vi "SetOutSumvGainAndOffset.vi"(6 "time out":u32, 9 "Real1":dbl, 10 "类型":u32(ring)=4 items=["PCI5121"=1, "PCI9810"=2, "USBCAN1"=3, "USBCAN2"=4, "PCI9820"=5, "CAN232"=6, "PCI5110"=7, "CANLite(mini)"=8, "ISA9620"=9, "ISA5420"=10, "PC104CAN"=11, "CANET"=17, "DNP9810"=13, "USBCAN-E-U"=20, "USBCAN-2E-U"=21], 11 "Real2":dbl, 12 "设备索引":u32(ring) items=["0", "1", "2", "3", "4", "5", "6", "7", "8", "9", "10", "11", "12", "13", "14", "15", ""], 13 "AD1":u16, 15 "AD2":u16, 16 "CAN路数":u32(ring) items=["0", "1"]) -> (20 "set ok?":bool, 22 "Gain":u16, 23 "Offset":u32)   [LabVIEW 2013]
uses:
  AutoBurn/Settings/ControlCAN.dll
panel:
  out "VCI_CAN_OBJ_T":T1 {"ID" format="%x"}
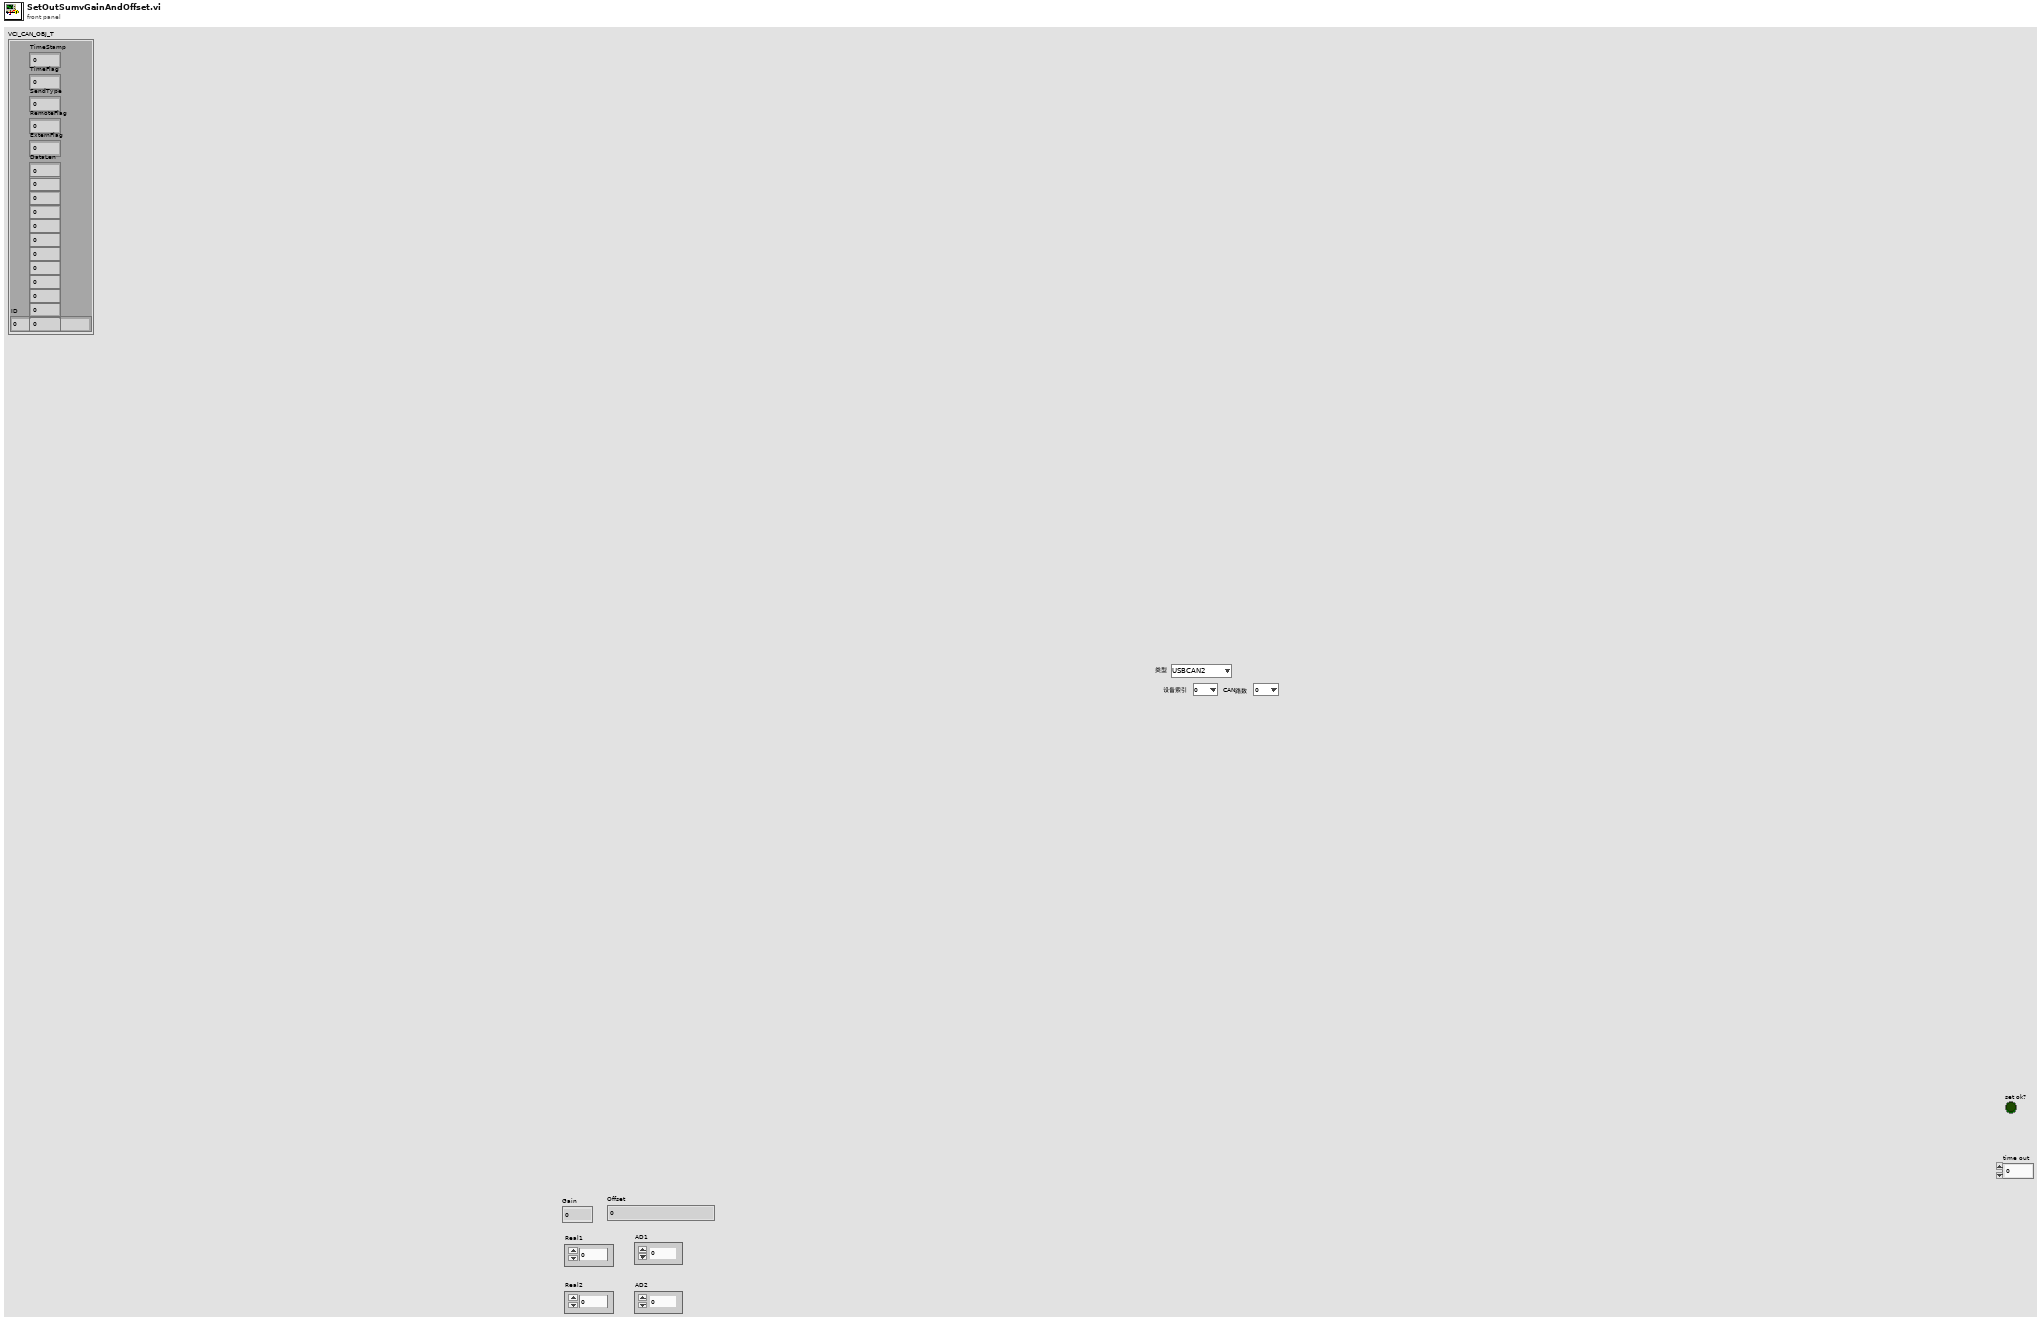
[diagram p1: front panel]
types:
  T1 = cluster{"ID":u32, "TimeStamp":u32, "TimeFlag":u8, "SendType":u8, "RemoteFlag":u8, "ExternFlag":u8, "DataLen":u8, u8, u8, u8, u8, u8, u8, u8, u8, u8, u8, u8}
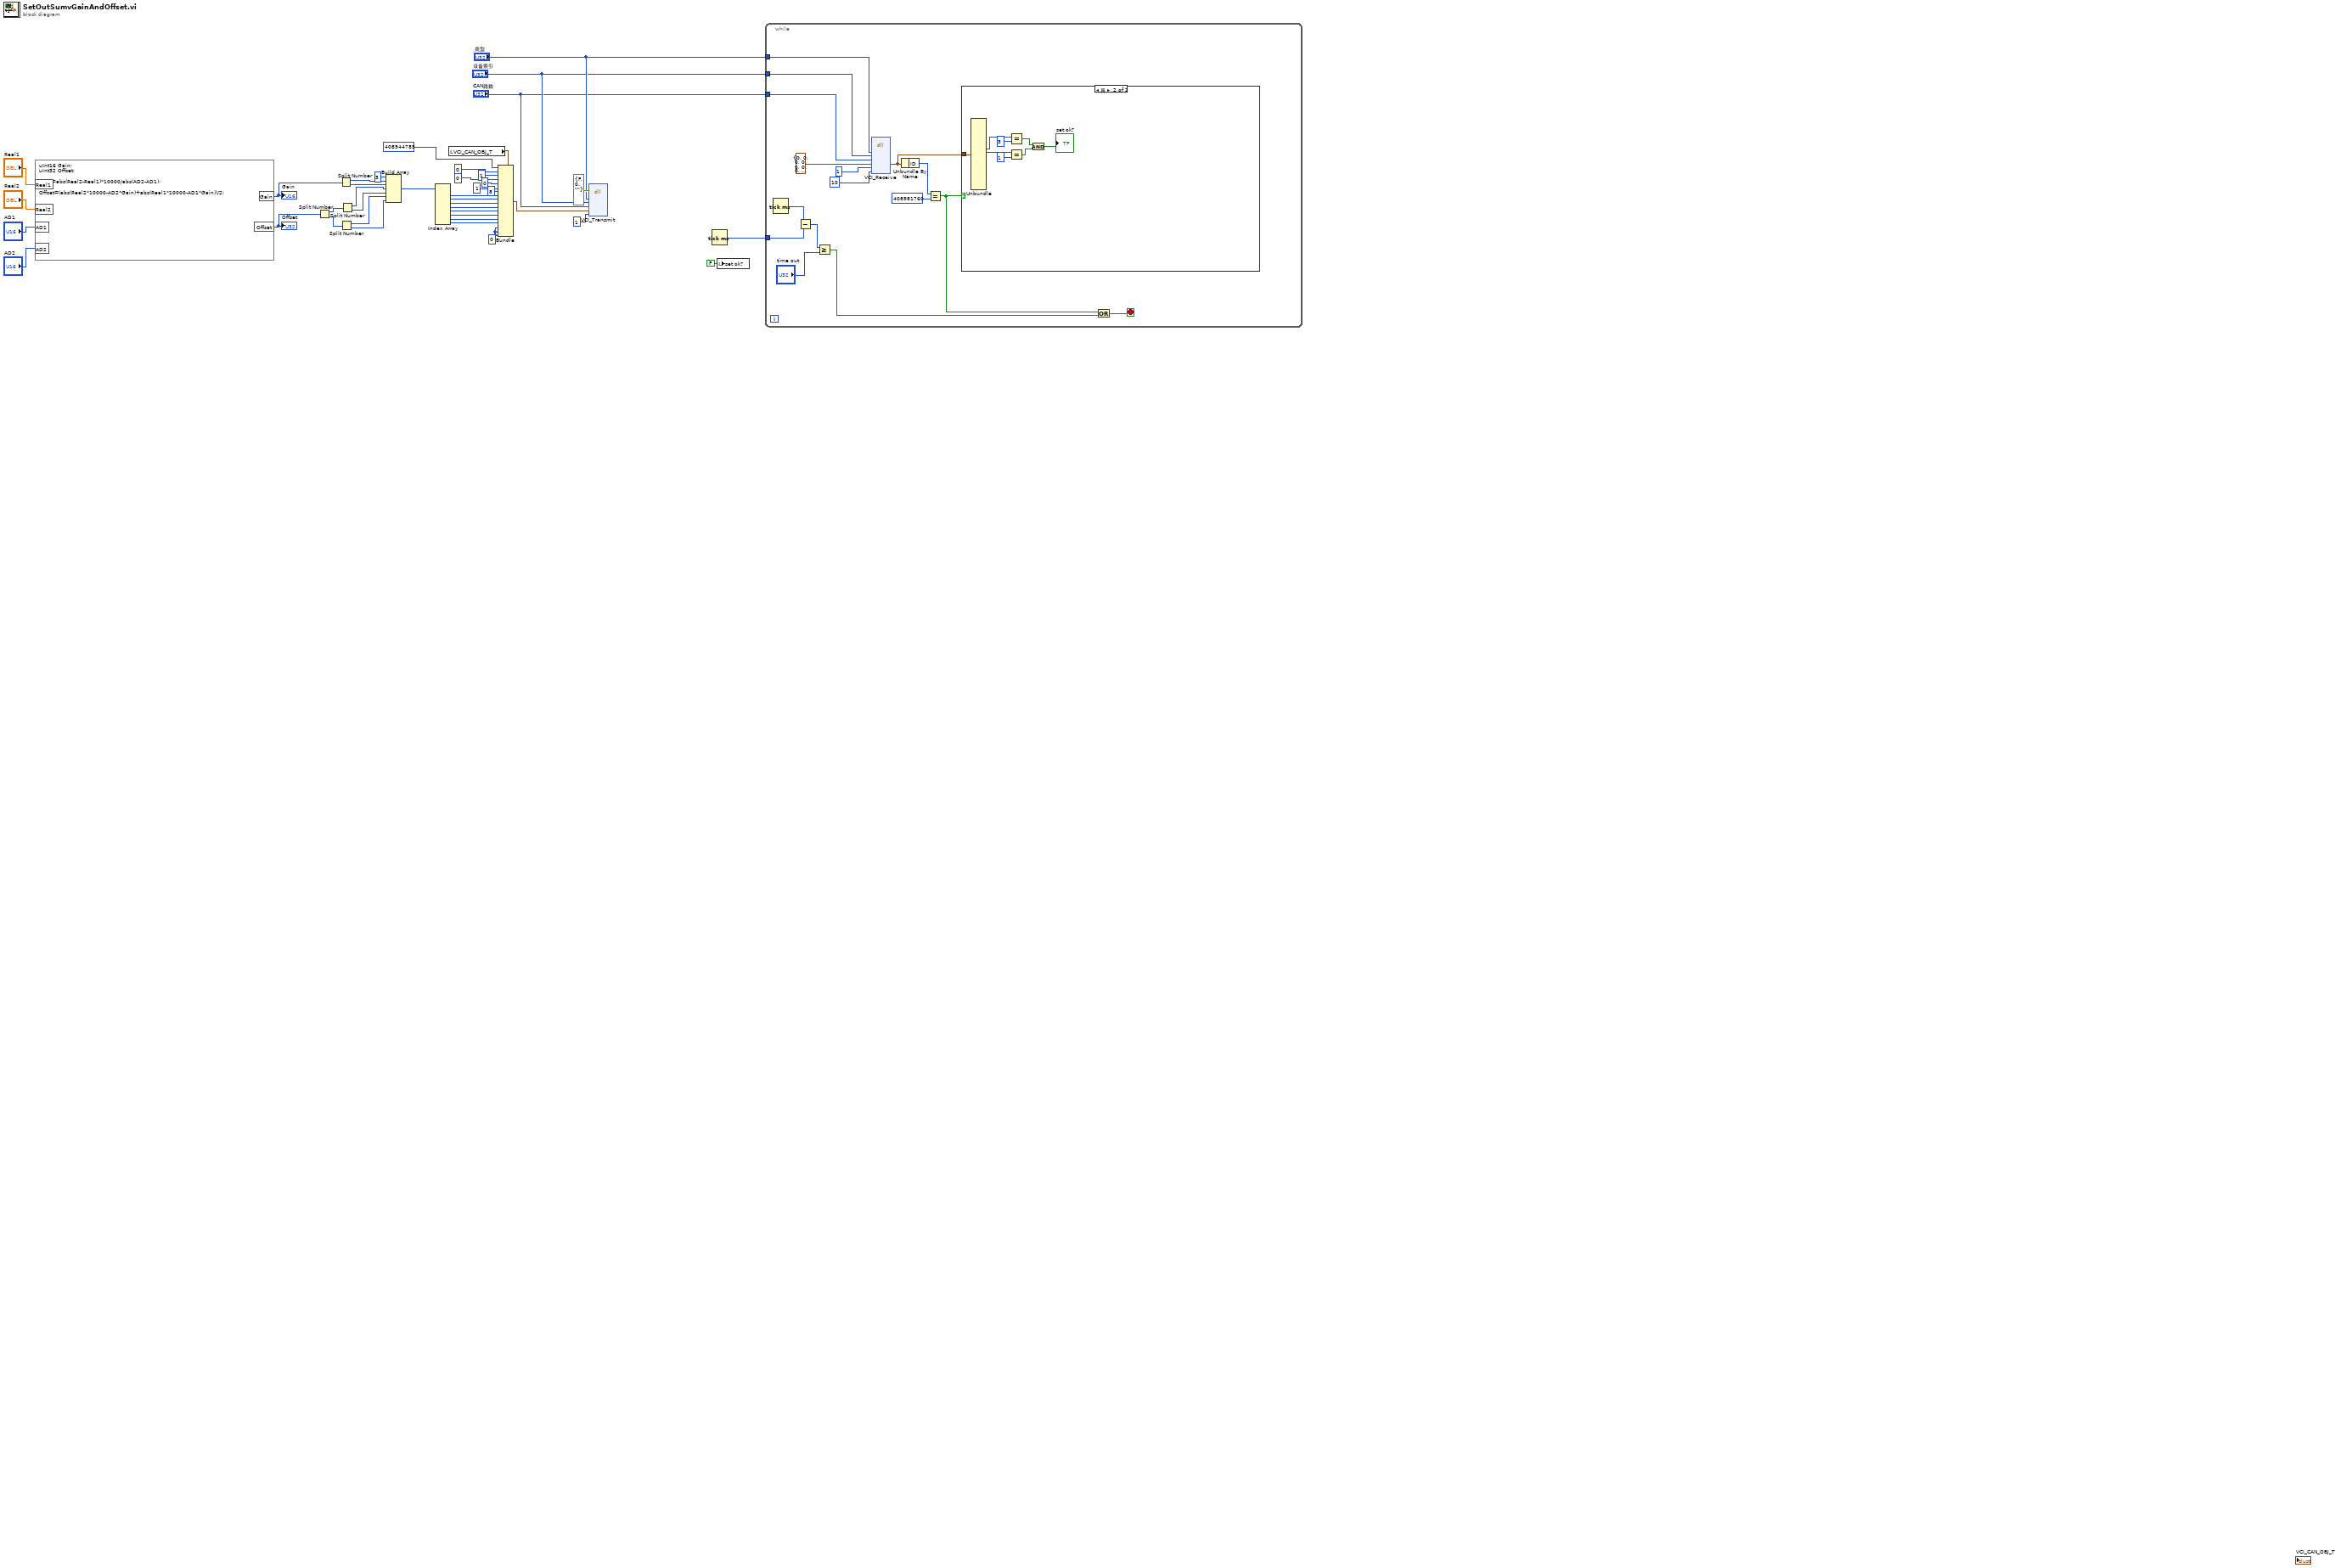
[diagram p0: block diagram]
diagram:
  w33 = u8 0 ("元素")
  n1 = formula code="uInt16 Gain;\nuInt32 Offset;\n\nGain=abs(Real2-Real1)*10000/abs(AD2-AD1);\n\nOffset=(abs(Real2*10000-AD2*Gain)+abs(Real1*10000-AD1*Gain))/2;"("Real1"="Real1", "Real2"="Real2", "AD1"="AD1", "AD2"="AD2") -> ("Gain"=w12:u16, "Offset"=w11:u32)
  "Gain" <- w12
  "Offset" <- w11
  n2 = Split Number(x=w11) -> (hi(x)=w10:u16, lo(x)=w9:u16)
  n3 = Split Number(x=w12) -> (hi(x)=w8:u8, lo(x)=w7:u8)
  n4 = Split Number(x=w9) -> (hi(x)=w4:u8, lo(x)=w3:u8)
  n5 = Split Number(x=w10) -> (hi(x)=w6:u8, lo(x)=w5:u8)
  n6 = Build Array(u8 3 ("元素"), w8, w7, w6, w5, w4, w3) -> (w1:u8[])
  n7 = Index Array(array=w1) -> (element #1=w31:u8, element #2=w30:u8, element #3=w29:u8, element #4=w28:u8, element #5=w27:u8, element #6=w26:u8, element #7=w25:u8, element #8=w24:u8)  [unwired: 8 in]
  n8 = local read "VCI_CAN_OBJ_T"() -> (w37:T1)
  n9 = Bundle(cluster=w37, "ID"=u32 408944785 ("RemoteFlag"), "TimeStamp"=u8 0 ("RemoteFlag"), "TimeFlag"=u8 1, "SendType"=u8 0 ("DataLen"), "RemoteFlag"=u8 0, "ExternFlag"=u8 1, "DataLen"=u8 8, w31, w30, w29, w28, w27, w26, w25, w24, w33, w33, w33) -> (w38:T1)
  n10 = dll-call lib="F:/Bluewave New Energy/SVN_Work/AutoTest_TestStand/trunk/AutoTest_TestStand/Driver/ZlgCan/BHN01/AutoBurn/Settings/ControlCAN.dll" fn="VCI_Transmit"(error in=errorcluster {"status"=FALSE, "code"=0, "source"=""} ("错误输入（无错误）"), "DeviceType"="类型", "DeviceInd"="设备索引", "CANInd"="CAN路数", "pSend"=w38, "Len"=u32 1) -> ()  [unwired: 4 in, 6 out]
  n11 = Tick Count (ms)() -> (millisecond timer value=w41:u32)
  n12 = local write "set ok?"(FALSE ("x = y?")) -> ()
  n13 = while {
    tunnel: w41 -> [w53]
    tunnel: "类型" -> [w44]
    tunnel: "设备索引" -> [w43]
    tunnel: "CAN路数" -> [w42]
    stop <- w47 stop-if-true
    n14 = Tick Count (ms)() -> (millisecond timer value=w54:u32)
    n15 = Subtract(x=w54, y=w53) -> (x-y=w52:u32)
    n16 = Greater Or Equal?(x=w52, y="time out") -> (x >= y?=w48:bool)
    n17 = dll-call lib="F:/Bluewave New Energy/SVN_Work/AutoTest_TestStand/trunk/AutoTest_TestStand/Driver/ZlgCan/BHN01/AutoBurn/Settings/ControlCAN.dll" fn="VCI_Receive"("DeviceType"=w44, "DeviceInd"=w43, "CANInd"=w42, "pReceive"=T1 {"ID"=0, "TimeStamp"=0, "TimeFlag"=0, "SendType"=0, "RemoteFlag"=0, "ExternFlag"=0, "DataLen"=0, 0, 0, 0, 0, 0, 0, 0, 0, 0, 0, 0}, "Len"=u32 1, "WaitTime"=10) -> ("pReceive"=w46:T1)  [unwired: 8 in, 3 out]
    n18 = Unbundle By Name(w46) -> ("ID"=w50:u32)
    n19 = Equal?(x=w50, y=u32 408981760) -> (x = y?=w49:bool)
    n20 = case shown="真" w49 {
      tunnel: w46 -> [_ w65]
      frame False {
      }
      frame True {
        n21 = Unbundle(w65) -> (w61:u8, w64:u8)  [unwired: 16 out]
        n22 = Equal?(x=w61, y=u8 3) -> (x = y?=w60:bool)
        n23 = Equal?(x=w64, y=u8 1) -> (x = y?=w59:bool)
        n24 = And(x=w60, y=w59) -> (x .and. y?=→"set ok?":bool)
      }
    }
    n25 = Or(x=w49, y=w48) -> (x .or. y?=w47:bool)
  }
